vi "Pneumatics Config.vi"(8 "error in (no error)":errorcluster, 11 "FileConfig in":refnum<class "FileConfig.lvclass">) -> (0 "error out":errorcluster, 1 "IDs found?":bool, 2 "Pneumatics Data":T1, 3 "FileConfig out":refnum<class "FileConfig.lvclass">, 5 "File Found?":bool)   [LabVIEW 2019, in "Config.lvlib" / "FileConfig.lvclass"]
doc: "Use this VI to get the IDs for the pneumatics of the robot."
uses:
  FileConfig.lvclass
  Config/Controls/Pneumatics Data.ctl
  <vilib>/Rock Robotics/WPI/Solenoid/WPI_SolenoidChannel.ctl
  FileConfig.lvclass/FileConfig.ctl
  Config.lvclass
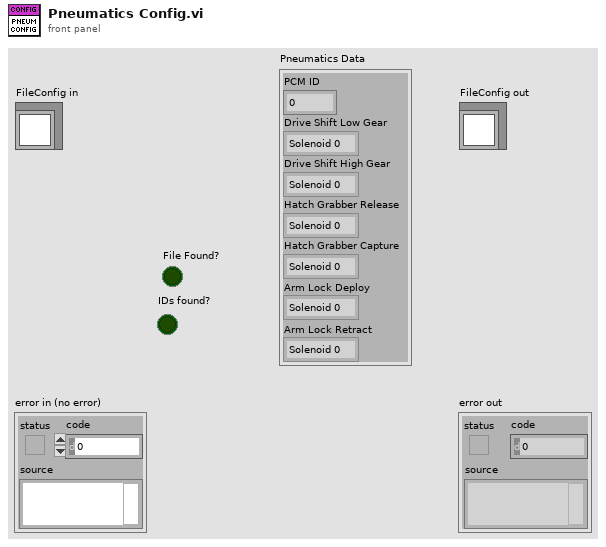
[diagram p1: front panel]
types:
  T1 = typedef "Config.lvlib/Config.lvclass/Pneumatics Data.ctl" = cluster{"PCM ID":u8, "Drive Shift Low Gear":T2, "Drive Shift High Gear":T2, "Hatch Grabber Release":T2, "Hatch Grabber Capture":T2, "Arm Lock Deploy":T2, "Arm Lock Retract":T2}
  T2 = typedef "WPI_SolenoidChannel.ctl" = enum8{"Solenoid 0", "Solenoid 1", "Solenoid 2", "Solenoid 3", "Solenoid 4", "Solenoid 5", "Solenoid 6", "Solenoid 7", "Invalid"}
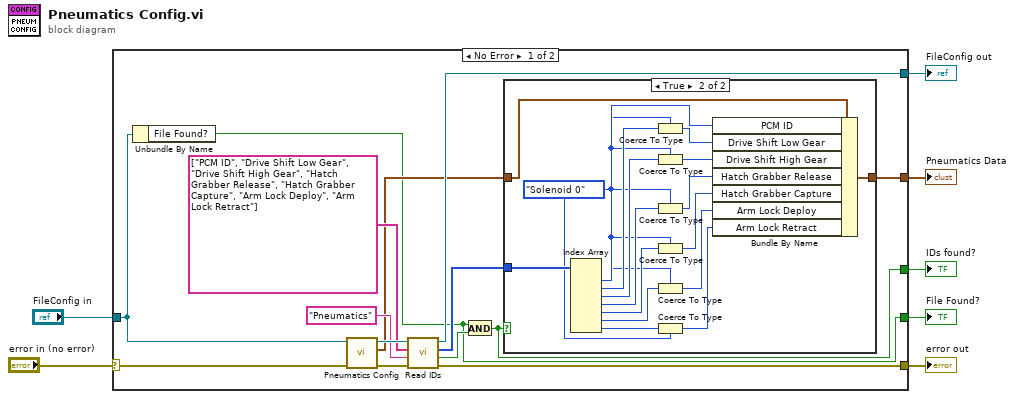
[diagram p0: block diagram]
diagram:
  n1 = case shown="No Error" "error in (no error)" {
    selector: "error in (no error)" -> [w20 w41]
    tunnel: [w19 w41] -> w7
    tunnel: [w13 _] -> w6
    tunnel: [w12 _] -> w5
    tunnel: [w17 w40] -> w4
    tunnel: [w8 _] -> w3
    tunnel: "FileConfig in" -> [w9 w40]
    frame No Error {
      n2 = Unbundle By Name(w9) -> ("File Found?"=w8:bool)
      n3 = call-parent "Pneumatics Config.vi"("error in (no error)"=w20, "Config in"=w9) -> ("error out"=w21:errorcluster, "Pneumatics Data"=w11:T1, "Config out"=w18:refnum<class "FileConfig.lvclass">)  [unwired: 5 in, 2 out]
      n4 = call "Read IDs.vi"("error in (no error)"=w21, "section"="Pneumatics", "keys"=string[] ["PCM ID", "Drive Shift Low Gear", "Drive Shift High Gear", "Hatch Grabber Release", "Hatch Grabber Capture", "Arm Lock Deploy", "Arm Lock Retract"], "FileConfig in"=w18) -> ("error out"=w19:errorcluster, "Found?"=w14:bool, "Found IDs"=w10:u8[], "FileConfig out"=w17:refnum<class "FileConfig.lvclass">)  [unwired: 4 in]
      n5 = And(x=w8, y=w14) -> (x .and. y?=w13:bool)
      n6 = case shown="True" w13 {
        tunnel: [w22 w38] -> w12
        tunnel: w11 -> [w22 w39]
        tunnel: w10 -> [_ w37]
        frame False {
        }
        frame True {
          w23 = WPI_SolenoidChannel."Solenoid 0" ("Forward Solenoid Channel")
          n7 = Index Array(array=w37) -> (element #1=w36:u8, element #2=w35:u8, element #3=w33:u8, element #4=w34:u8, element #5=w32:u8, element #6=w26:u8, element #7=w25:u8)  [unwired: 7 in]
          n8 = Coerce To Type(0:w35, 1:w23) -> (2:w28:T2)
          n9 = Coerce To Type(0:w33, 1:w23) -> (2:w29:T2)
          n10 = Coerce To Type(0:w34, 1:w23) -> (2:w30:T2)
          n11 = Coerce To Type(0:w32, 1:w23) -> (2:w31:T2)
          n12 = Coerce To Type(0:w26, 1:w23) -> (2:w27:T2)
          n13 = Coerce To Type(0:w25, 1:w23) -> (2:w24:T2)
          n14 = Bundle By Name(cluster=w39, "PCM ID"=w36, "Drive Shift Low Gear"=w28, "Drive Shift High Gear"=w29, "Hatch Grabber Release"=w30, "Hatch Grabber Capture"=w31, "Arm Lock Deploy"=w27, "Arm Lock Retract"=w24) -> (w38:T1)
        }
      }
    }
    frame Error {
    }
  }
  "error out" <- w7
  "FileConfig out" <- w4
  "File Found?" <- w3
  "IDs found?" <- w6
  "Pneumatics Data" <- w5
